vi "Настройка и измерение мультиметром 34980A.vi"(0 "Коммутатор Agilent 34980A in":refnum<visa-resource-name>, 11 "error in":errorcluster, 12 "Скорост измерения":u16(ring) items=["1NPLC", "10 NPLC"], 13 "Число измерений":i32=1) -> (4 "Коммутатор Agilent 34980A out":refnum<visa-resource-name>, 6 "+U /-U выходное":dbl[](array[numeric]), 15 "error out 2":errorcluster)   [LabVIEW 2017]
uses:
  <instrlib>/niDMM/nidmm.llb/niDMM Function.ctl
  <instrlib>/niDMM/nidmm.llb/niDMM Auto Zero.ctl
  <instrlib>/niDMM/nidmm.llb/niDMM ADC Calibration.ctl
  <instrlib>/niDMM/nidmm.llb/niDMM Configure Measurement Absolute.vi
panel:
  out "error out":errorcluster
  out "Aperture Time":dbl format="%.2p"
  out "x-y":u32
  out "x*y":dbl
  in  "Number to Read":i32=1000
  out "Measurement Period (seconds) 2":dbl caption="Measurement Period (seconds)" format="%.4f"
  in  "Numeric":i32
  out "Measurements":dbl[](array[numeric]) format="%.2f"
  out "Measurement Period (seconds)":dbl format="%.4f"
  in  "ADC Calibration":T1=-1 items=["Auto"=-1, "Off"=0, "On"=1]
  in  "Auto Zero":T2=-1 items=["Auto"=-1, "Off"=0, "On"=1, "Once"=2]
  in  "Range":dbl=0.02 format="%.2f"
  in  "Function":T3
  in  "Resolution":dbl=0.001 format="%.5f"
  in  "Instrument Descriptor":refnum<k15>
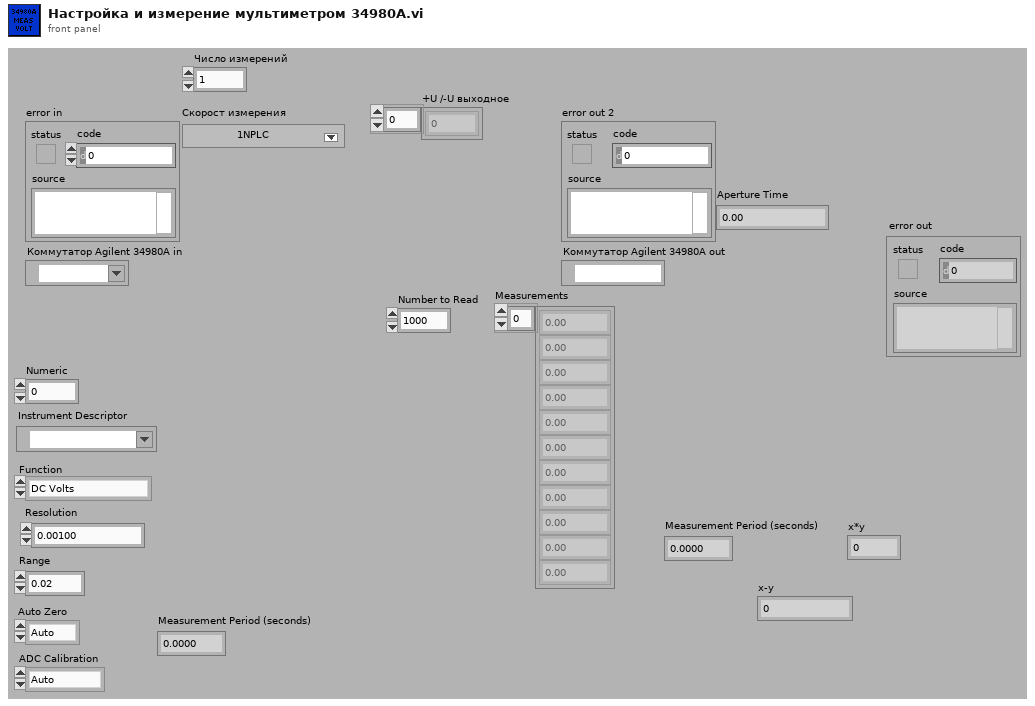
[diagram p1: front panel]
types:
  T1 = typedef "niDMM ADC Calibration.ctl" = i32
  T2 = typedef "niDMM Auto Zero.ctl" = i32
  T3 = typedef "niDMM Function.ctl" = enum16{"DC Volts", "AC Volts", "DC Current", "AC Current", "2-wire Resistance", "4-wire Resistance", "Diode", "Frequency", "Period", "AC Volts DC Coupled", "Capacitance", "Inductance", "Temperature"}
  T4 = enum16{"0.02 PLC", "0.2 PLC", "1 PLC", "2 PLC", "10 PLC", "20 PLC", "100 PLC", "200 PLC"}
  T5 = enum16{"4 1/2", "5 1/2", "6 1/2", "Least", "Highest", "Default"}
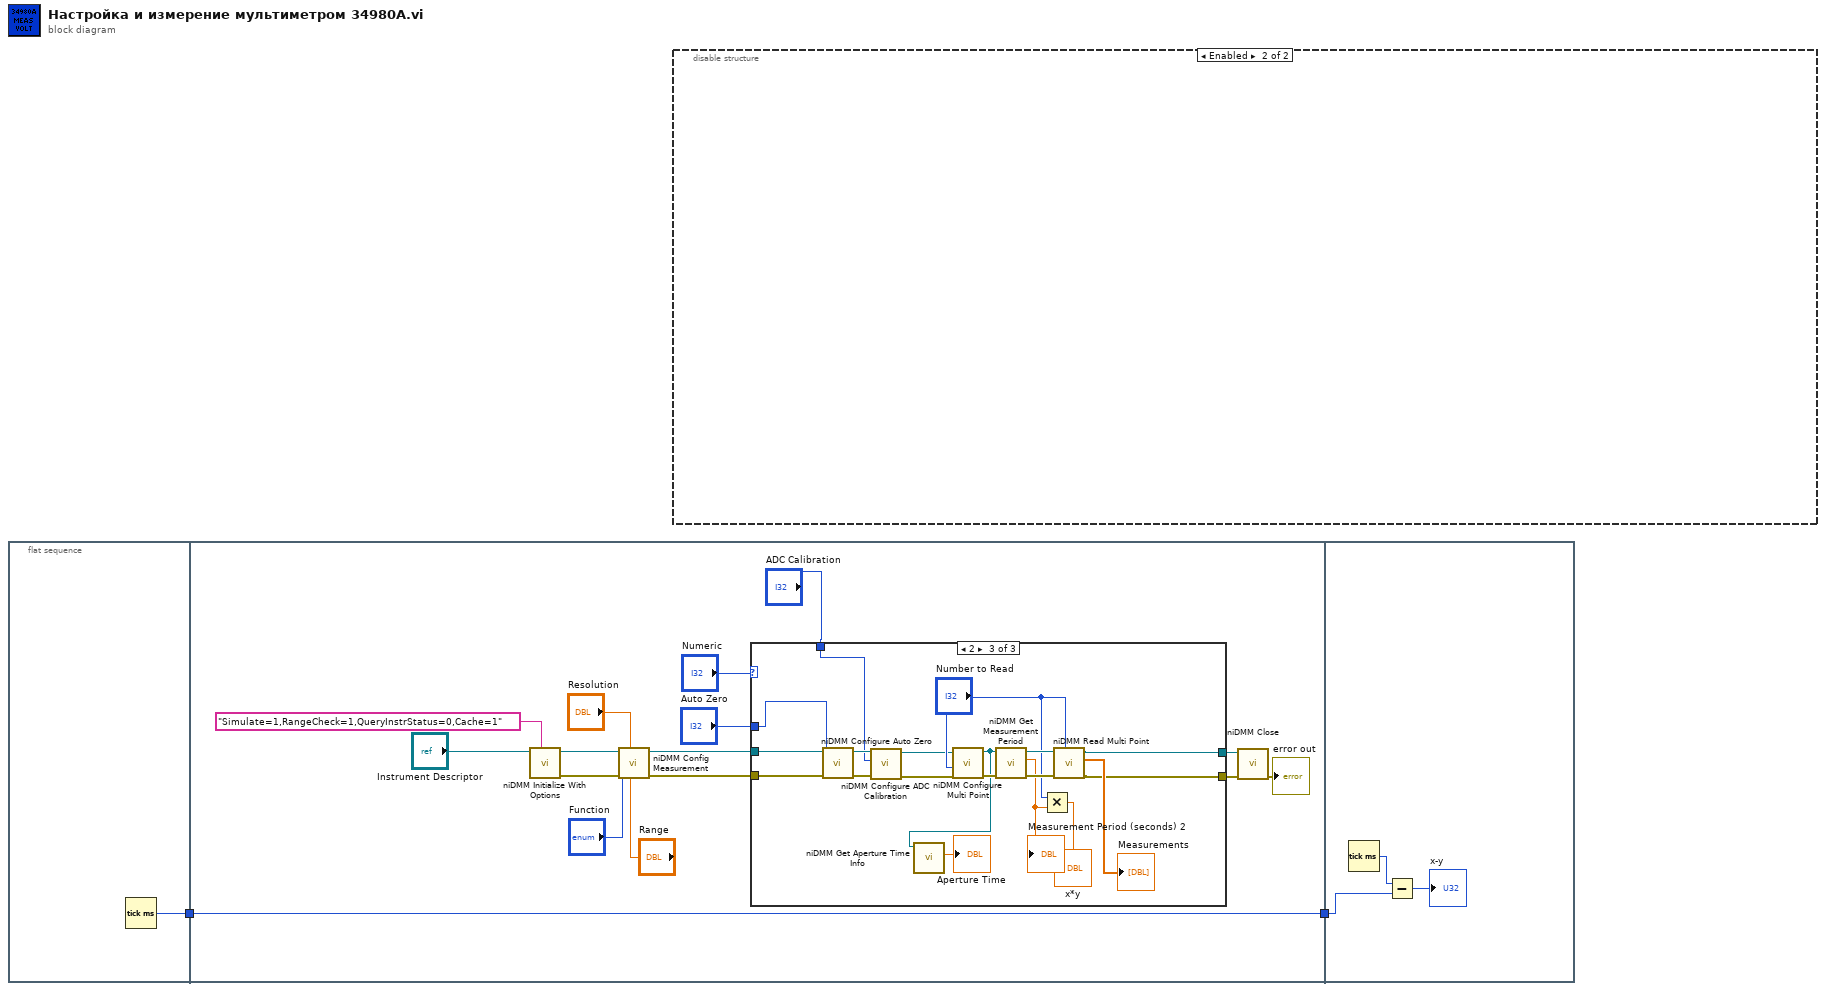
[diagram p0: block diagram]
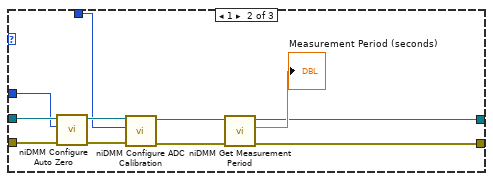
[diagram p3: hidden frame]
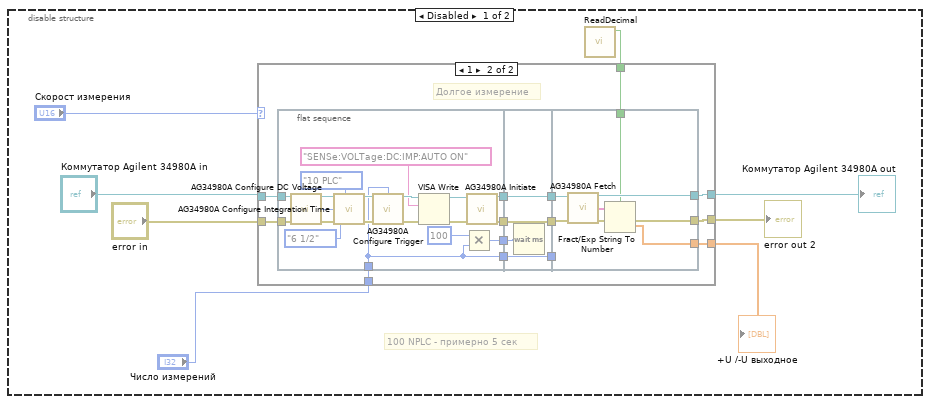
[diagram p4: hidden frame]
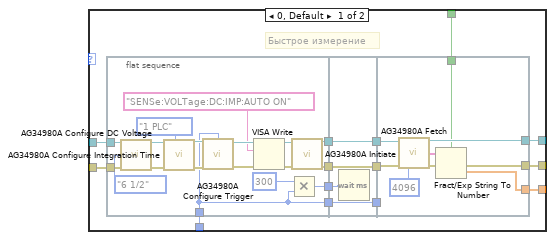
[diagram p5: hidden frame]
diagram:
  n1 = flat-sequence {
    tunnel: [w3] -> w2
    tunnel: w2 -> [w5]
    tunnel: [w5] -> w1
    tunnel: w1 -> [w53]
    frame #0 {
      n2 = Tick Count (ms)() -> (millisecond timer value=w3:u32)
    }
    frame #1 {
      n3 = call <instrlib>:"niDMM Initialize With Options.vi"("Option String"="Simulate=1,RangeCheck=1,QueryInstrStatus=0,Cache=1", "Instrument Descriptor"="Instrument Descriptor") -> ("error out"=w17:errorcluster, "instrument handle out"=w16:refnum<k15>)  [unwired: 8 in]
      n4 = call-poly <instrlib>:"niDMM Config Measurement.vi"("Range"="Range", "Resolution"="Resolution", "error in (no error)"=w17, "Function"="Function", "instrument handle"=w16) -> ("error out"=w11:errorcluster, "instrument handle out"=w12:refnum<k15>)  [unwired: 5 in]
      n5 = case shown="2" "Numeric" {
        tunnel: w12 -> [w21 w32 w50]
        tunnel: w11 -> [w20 w31 w49]
        tunnel: [w20 w25 w43] -> w10
        tunnel: [w21 w24 w44] -> w9
        tunnel: "Auto Zero" -> [_ w23 w48]
        tunnel: "ADC Calibration" -> [_ w22 w36]
        frame 0, Default {
        }
        frame 1 {
          n6 = call <instrlib>:"niDMM Configure Auto Zero.vi"("error in (no error)"=w31, "Auto Zero"=w23, "instrument handle"=w32) -> ("error out"=w29:errorcluster, "instrument handle out"=w30:refnum<k15>)  [unwired: 7 in]
          n7 = call <instrlib>:"niDMM Configure ADC Calibration.vi"("error in (no error)"=w29, "ADC Calibration"=w22, "instrument handle"=w30) -> ("error out"=w28:errorcluster, "instrument handle out"=w27:refnum<k15>)  [unwired: 7 in]
          n8 = call <instrlib>:"niDMM Get Measurement Period.vi"("error in (no error)"=w28, "instrument handle"=w27) -> ("error out"=w25:errorcluster, "Measurement Period (seconds)"=→"Measurement Period (seconds)":dbl, "instrument handle out"=w24:refnum<k15>)  [unwired: 7 in]
        }
        frame 2 {
          n9 = call <instrlib>:"niDMM Configure Auto Zero.vi"("error in (no error)"=w49, "Auto Zero"=w48, "instrument handle"=w50) -> ("error out"=w38:errorcluster, "instrument handle out"=w39:refnum<k15>)  [unwired: 7 in]
          n10 = call <instrlib>:"niDMM Configure ADC Calibration.vi"("error in (no error)"=w38, "ADC Calibration"=w36, "instrument handle"=w39) -> ("error out"=w37:errorcluster, "instrument handle out"=w35:refnum<k15>)  [unwired: 7 in]
          n11 = call <instrlib>:"niDMM Configure Multi Point.vi"("error in (no error)"=w37, "Sample Count"="Number to Read", "instrument handle"=w35) -> ("error out"=w47:errorcluster, "instrument handle out"=w33:refnum<k15>)  [unwired: 7 in]
          n12 = call <instrlib>:"niDMM Get Aperture Time Info.vi"("instrument handle"=w33) -> ("Aperture Time"=→"Aperture Time":dbl)  [unwired: 7 in, 3 out]
          n13 = call <instrlib>:"niDMM Get Measurement Period.vi"("error in (no error)"=w47, "instrument handle"=w33) -> ("error out"=w45:errorcluster, "Measurement Period (seconds)"=w41:dbl, "instrument handle out"=w46:refnum<k15>)  [unwired: 7 in]
          "Measurement Period (seconds) 2" <- w41
          n14 = Multiply(x="Number to Read", y=w41) -> (x*y=→"x*y":dbl)
          n15 = call <instrlib>:"niDMM Read Multi Point.vi"("Number to Read"="Number to Read", "error in (no error)"=w45, "instrument handle"=w46) -> ("error out"=w43:errorcluster, "Measurements"=→"Measurements":dbl[], "instrument handle out"=w44:refnum<k15>)  [unwired: 5 in, 1 out]
        }
      }
      n16 = call <instrlib>:"niDMM Close.vi"("error in (no error)"=w10, "instrument handle"=w9) -> ("error out"=→"error out":errorcluster)  [unwired: 9 in]
    }
    frame #2 {
      n17 = Tick Count (ms)() -> (millisecond timer value=w54:u32)
      n18 = Subtract(x=w54, y=w53) -> (x-y=→"x-y":u32)
    }
  }
  n19 = disable-structure shown="Enabled" {
    frame Disabled {
      # "100 NPLC - примерно 5 сек"
      n20 = call "ReadDecimal.vi"() -> ("Флаг Разделителя"=w55:bool)  [unwired: 11 in]
      n21 = case shown="1" "Скорост измерения" {
        tunnel: "Коммутатор Agilent 34980A in" -> [w76 w120]
        tunnel: "error in" -> [w75 w119]
        tunnel: [w69 w113] -> w60
        tunnel: [w70 w114] -> w59
        tunnel: [w64 w108] -> w56
        tunnel: "Число измерений" -> [w68 w112]
        tunnel: w55 -> [w63 w107]
        frame 0, Default {
          # "Быстрое измерение"
          n22 = flat-sequence {
            tunnel: w76 -> [w94]
            tunnel: w75 -> [w93]
            tunnel: [w88] -> w74
            tunnel: [w87] -> w73
            tunnel: w68 -> [w82]
            tunnel: [w83] -> w67
            tunnel: [w82] -> w66
            tunnel: w74 -> [w98]
            tunnel: w73 -> [w97]
            tunnel: [w98] -> w72
            tunnel: [w97] -> w71
            tunnel: w67 -> [w96]
            tunnel: w66 -> [w95]
            tunnel: [w95] -> w65
            tunnel: w72 -> [w106]
            tunnel: w71 -> [w103]
            tunnel: [w105] -> w70
            tunnel: [w104] -> w69
            tunnel: w65 -> [_]
            tunnel: [w99] -> w64
            tunnel: w63 -> [w100]
            frame #0 {
              n23 = call "AG34980A Configure DC Voltage.vi"("VISA resource name"=w94, "Resolution (5:Default)"=T5."6 1/2", "error in (no error)"=w93) -> ("VISA resource name out"=w90:refnum<visa-resource-name>, "error out"=w91:errorcluster)  [unwired: 11 in]
              n24 = call "AG34980A Configure Integration Time.vi"("NPLC Value(6:1PLC)"=T4."1 PLC", "error in (no error)"=w91, "VISA resource name"=w90) -> ("error out"=w85:errorcluster, "VISA resource name out"=w86:refnum<visa-resource-name>)  [unwired: 7 in]
              n25 = call "AG34980A Configure Trigger.vi"("VISA resource name"=w86, "Sample Count (1)"=w82, "error in (no error)"=w85) -> ("VISA resource name out"=w79:refnum<visa-resource-name>, "error out"=w78:errorcluster)  [unwired: 11 in]
              n26 = VISA Write(VISA resource name=w79, write buffer="SENSe:VOLTage:DC:IMP:AUTO ON", error in (no error)=w78) -> (VISA resource name out=w81:refnum<visa-resource-name>, error out=w80:errorcluster)  [unwired: 1 out]
              n27 = Multiply(x=300, y=w82) -> (x*y=w83:i32)
              n28 = call "AG34980A Initiate.vi"("VISA resource name"=w81, "error in (no error)"=w80) -> ("VISA resource name out"=w88:refnum<visa-resource-name>, "error out"=w87:errorcluster)  [unwired: 12 in]
            }
            frame #1 {
              n29 = Wait (ms)(milliseconds to wait=w96) -> ()  [unwired: 1 out]
            }
            frame #2 {
              n30 = call "AG34980A Fetch.vi"("VISA resource name"=w106, "error in (no error)"=w103, "Byte Count (1024 bytes)"=4096) -> ("VISA resource name out"=w105:refnum<visa-resource-name>, "Output Data"=w102:string[], "error out"=w104:errorcluster)  [unwired: 9 in, 1 out]
              n31 = Fract/Exp String To Number(use system decimal point (T)=w100, string=w102) -> (number=w99:dbl[])  [unwired: 2 in, 1 out]
            }
          }
        }
        frame 1 {
          # "Долгое измерение"
          n32 = flat-sequence {
            tunnel: w120 -> [w138]
            tunnel: w119 -> [w137]
            tunnel: [w132] -> w118
            tunnel: [w131] -> w117
            tunnel: w112 -> [w126]
            tunnel: [w127] -> w111
            tunnel: [w126] -> w110
            tunnel: w118 -> [w142]
            tunnel: w117 -> [w141]
            tunnel: [w142] -> w116
            tunnel: [w141] -> w115
            tunnel: w111 -> [w140]
            tunnel: w110 -> [w139]
            tunnel: [w139] -> w109
            tunnel: w116 -> [w149]
            tunnel: w115 -> [w146]
            tunnel: [w148] -> w114
            tunnel: [w147] -> w113
            tunnel: w109 -> [_]
            tunnel: [w143] -> w108
            tunnel: w107 -> [w144]
            frame #0 {
              n33 = call "AG34980A Configure DC Voltage.vi"("VISA resource name"=w138, "Resolution (5:Default)"=T5."6 1/2", "error in (no error)"=w137) -> ("VISA resource name out"=w134:refnum<visa-resource-name>, "error out"=w135:errorcluster)  [unwired: 11 in]
              n34 = call "AG34980A Configure Integration Time.vi"("NPLC Value(6:1PLC)"=T4."10 PLC", "error in (no error)"=w135, "VISA resource name"=w134) -> ("error out"=w129:errorcluster, "VISA resource name out"=w130:refnum<visa-resource-name>)  [unwired: 7 in]
              n35 = call "AG34980A Configure Trigger.vi"("VISA resource name"=w130, "Sample Count (1)"=w126, "error in (no error)"=w129) -> ("VISA resource name out"=w123:refnum<visa-resource-name>, "error out"=w122:errorcluster)  [unwired: 11 in]
              n36 = VISA Write(VISA resource name=w123, write buffer="SENSe:VOLTage:DC:IMP:AUTO ON", error in (no error)=w122) -> (VISA resource name out=w124:refnum<visa-resource-name>, error out=w125:errorcluster)  [unwired: 1 out]
              n37 = Multiply(x=100, y=w126) -> (x*y=w127:i32)
              n38 = call "AG34980A Initiate.vi"("VISA resource name"=w124, "error in (no error)"=w125) -> ("VISA resource name out"=w132:refnum<visa-resource-name>, "error out"=w131:errorcluster)  [unwired: 12 in]
            }
            frame #1 {
              n39 = Wait (ms)(milliseconds to wait=w140) -> ()  [unwired: 1 out]
            }
            frame #2 {
              n40 = call "AG34980A Fetch.vi"("VISA resource name"=w149, "error in (no error)"=w146) -> ("VISA resource name out"=w148:refnum<visa-resource-name>, "Output Data"=w145:string[], "error out"=w147:errorcluster)  [unwired: 10 in, 1 out]
              n41 = Fract/Exp String To Number(use system decimal point (T)=w144, string=w145) -> (number=w143:dbl[])  [unwired: 2 in, 1 out]
            }
          }
        }
      }
      "error out 2" <- w60
      "Коммутатор Agilent 34980A out" <- w59
      "+U /-U выходное" <- w56
    }
    frame Enabled {
    }
  }
